vi "Logowanie_alternatywny_lepszy_sposob.vi"() -> ()   [LabVIEW 2012]
panel:
  out "zaloguj":bool
  out "haslo":string
  out "login":string
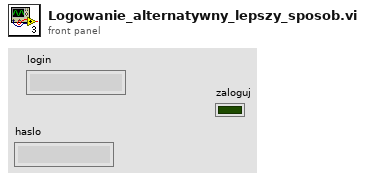
[diagram p1: front panel]
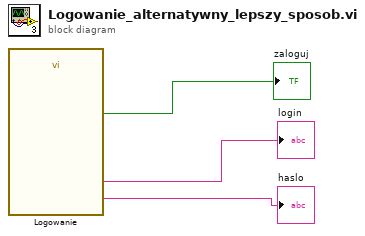
[diagram p0: block diagram]
diagram:
  n1 = call "Logowanie"() -> ("Podaj hasło:"=→"haslo":string, "Podaj nazwę:"=→"login":string, "Dalej"=→"zaloguj":bool)  [unwired: 16 in, 1 out]
